vi "Modify CE template to Single point CE template.vi"(8 "error in (no error)":errorcluster, 10 "Measurement template file":path, 11 "SS measurement":T1 {"PJVS reference voltages array of vector cluster"."PJVS reference voltages vector" format="%#_3p"; "PJVS frequencies (Hz)" format="%#_3p"; "Record lengths (multiples of periods)" format="%#_3p"; "Sampling frequencies (Hz)" format="%#_3p"; "Signal amplitudes (V)" format="%#_3p"; "Signal frequencies (Hz)" format="%#_3p"}) -> (0 "error out":errorcluster)   [LabVIEW 2020]
doc: "Modify CE template - set CE measurement for only one frequency, sets amplitude and sampling frequency, removes possible previous measured data."
uses:
  SS Measurement/Type definitions/SS measurement.ctl
  <vilib>/Utility/NIReport.llb/Report Type.ctl
  <vilib>/Utility/NIReport.llb/NI_report.lvclass
  <vilib>/Utility/NIReport.llb/NI_ReportGenerationCore.lvlib
  external libraries/varilib/varilib.lvlib
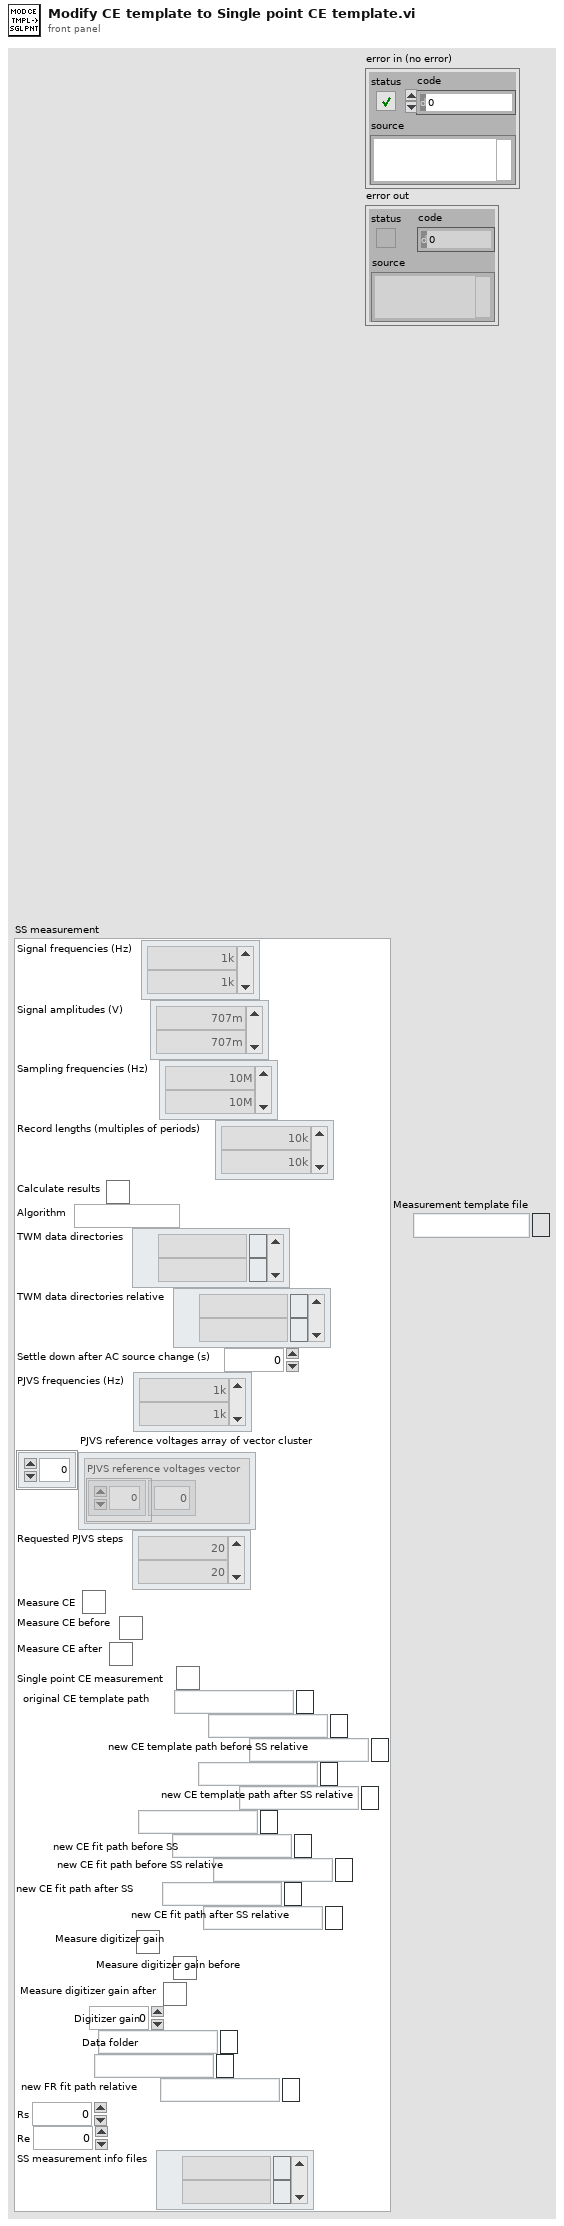
[diagram p1: front panel]
types:
  T1 = typedef "SS measurement.ctl" = cluster{"Signal frequencies (Hz)":dbl[], "Signal amplitudes (V)":dbl[], "Sampling frequencies (Hz)":dbl[], "Record lengths (multiples of periods)":dbl[], "Calculate results":bool, "Algorithm":string, "TWM data directories":path[], "TWM data directories relative":path[], "Settle down after AC source change (s)":dbl, "PJVS frequencies (Hz)":dbl[], "PJVS reference voltages array of vector cluster":cluster{"PJVS reference voltages vector":dbl[]}[], "Requested PJVS steps":u32[], "Measure CE":bool, "Measure CE before":bool, "Measure CE after":bool, "Single point CE measurement":bool, "original CE template path":path, "new CE template path before SS":path, "new CE template path before SS relative":path, "new CE template path after SS":path, "new CE template path after SS relative":path, "original CE fit path":path, "new CE fit path before SS":path, "new CE fit path before SS relative":path, "new CE fit path after SS":path, "new CE fit path after SS relative":path, "Measure digitizer gain":bool, "Measure digitizer gain before":bool, "Measure digitizer gain after":bool, "Digitizer gain":dbl, "Data folder":path, "FR fit path":path, "new FR fit path relative":path, "Rs":i32, "Re":i32, "SS measurement info files":path[]}
  T2 = typedef "NI_ReportGenerationCore.lvlib/Report Type.ctl" = enum16{"HTML", "Word", "Excel"}
  T3 = enum16{"maximized", "minimized", "normal", "no change"}
  T4 = typedef "Type definitions to be saved.ctl" = cluster{"Common properties":T5, "AC Source":T6, "DC meter":T8, "CE measurement":T10, "FR measurement":T11, "FR template":T12, "CE template":T13, "PJVS":T14, "SS measurement":T1, "AC sync source":T6}
  T5 = typedef "Common properties.ctl" = cluster{"Measurement status ref":refnum<vi>, "TWM Status ref":refnum<vi>, "Abort ref":refnum<vi>, "Skip waiting ref":refnum<vi>, "GNU Octave path":path, "TWM+QWTB path":path, "lvlib path":path, "TWM pipe":string, "PJVS status ref":refnum<vi>, "WAC path":path}
  T6 = typedef "AC Source.ctl" = cluster{"AC Source type":T7, "VISA":refnum<visa-resource-name>, "Ref. clock (Hz)":dbl, "status ref":refnum<vi>, "Fluke 57XX wideband output":bool, "Fluke 57XX ignore errors":bool, "Synchronization by AC signal":bool}
  T7 = typedef "AC Source type.ctl" = enum16{"Fluke 5XXX calibrator", "Tektronix AFG3000 series", "dummy", "Agilent 331xxA to 332xxA", "Agilent 335xxA to 336xxA"}
  T8 = typedef "DC meter.ctl" = cluster{"DC meter type":T9, "DC meter VISA":refnum<visa-resource-name>, "NPLC":dbl, "status ref":refnum<vi>}
  T9 = typedef "DC meter type.ctl" = enum16{"H/A/K 3458", "Fluke 8508A", "dummy", "Keithley 2182"}
  T10 = typedef "CE measurement.ctl" = cluster{"Signal frequencies (Hz) T":dbl[], "Signal amplitudes (V) T":dbl[], "Sampling frequencies (Hz) T":dbl[], "Record lengths (multiples of periods) T":dbl[], "TWM data root directory":path, "TWM mreasurements directories":path[], "Calculate RMS from samples":bool, "RMS algorithm T":string, "Settle down after AC source change (s) T":dbl, "Skip PJVS setup":bool, "Measurement template file":path, "Row of START keyword T":i32, "Row of STOP keyword T":i32, "Measurement template line T":i32[], "Switch position T":dbl[], "FR fit mat file T":path, "Recalculate-skip already calculated":bool}
  T11 = typedef "FR measuement.ctl" = cluster{"Measurement frequencies (Hz)":dbl[], "Sampling frequency (Hz)":dbl, "Signal amplitude (V)":dbl, "AC-DC settle time (s)":dbl, "Record length (multiples of period)":dbl[], "Measurement template file":path, "Row of START keyword":i32, "Row of STOP keyword":i32, "Calculate RMS from samples":bool, "AC-DC warm up time (s)":dbl, "Measurement template line":i32[], "DC meter readings No.":i32, "Algorithm":string, "Simultaneous measurement":bool, "Recalculate-skip already calculated":bool}
  T12 = typedef "FR template.ctl" = cluster{"Keywords column":i32, "Sig. freq. column":i32, "Rec. len. column":i32, "Meas. points. row min to read":i32, "Meas. points. row max to read":i32, "Properties column":i32, "Properties row start":i32, "Properties row end":i32, "Keyword START regexp":string, "Keyword STOP regexp":string, "HW data column":i32, "HW data row start":i32, "HW data row end":i32, "TIme and date column start":i32, "Digitizer value column start ":i32, "DC mean column start ":i32, "DC readings column start":i32}
  T13 = typedef "CE template.ctl" = cluster{"Keywords column":i32, "Sig. freq. column":i32, "Rec. len. column":i32, "Switch pos column":i32, "Meas. points. row min to read":i32, "Meas. points. row max to read":i32, "Properties column":i32, "Properties row start":i32, "Properties row end":i32, "Keyword START regexp":string, "Keyword STOP regexp":string, "HW data column":i32, "HW data row start":i32, "HW data row end":i32, "TIme and date column start":i32, "Digitizer value column start ":i32}
  T14 = typedef "PJVS.ctl" = cluster{"PJVS type":T15, "Status Refnum":refnum<vi>, "AC-supraVOLTcontrol":cluster{"IP address:port (0.0.0.0:0000)":string, "Timeouts":T16, "Simulation mode":bool, "Debug mode":bool}, "NPL bias source":cluster{"DataSocketCluster":T17}, "Manual PJVS":cluster{"PJVS frequency (Hz)":dbl, "Reference voltages (V)":dbl[], "File with PJVS voltages":path}, "VTT PJVS":cluster{"some VTT only property":string}}
  T15 = typedef "PJVS Type.ctl" = enum16{"AC-supraVOLTcontrol", "JV modified NPL bias control", "Manual PJVS", "VTT PJVS"}
  T16 = typedef "ACSVcontrol-driver.lvlib/Timeouts.ctl" = cluster{"TCP Read & Write (ms)":i32, "Sensors readout":i32, "PJVS setup":i32, "Nullmeter readout":i32, "Multiplexer setup":i32, "57XX setup":i32, "Generator setup":i32, "Synthesizer setup":i32, "Sampler readout":i32}
  T17 = typedef "DataSocketCluster external.ctl" = cluster{"Server Machine":string, "Client Machine":string, "Data":string, "TimeStamp":dbl, "Count":i32, "Target Process":string}
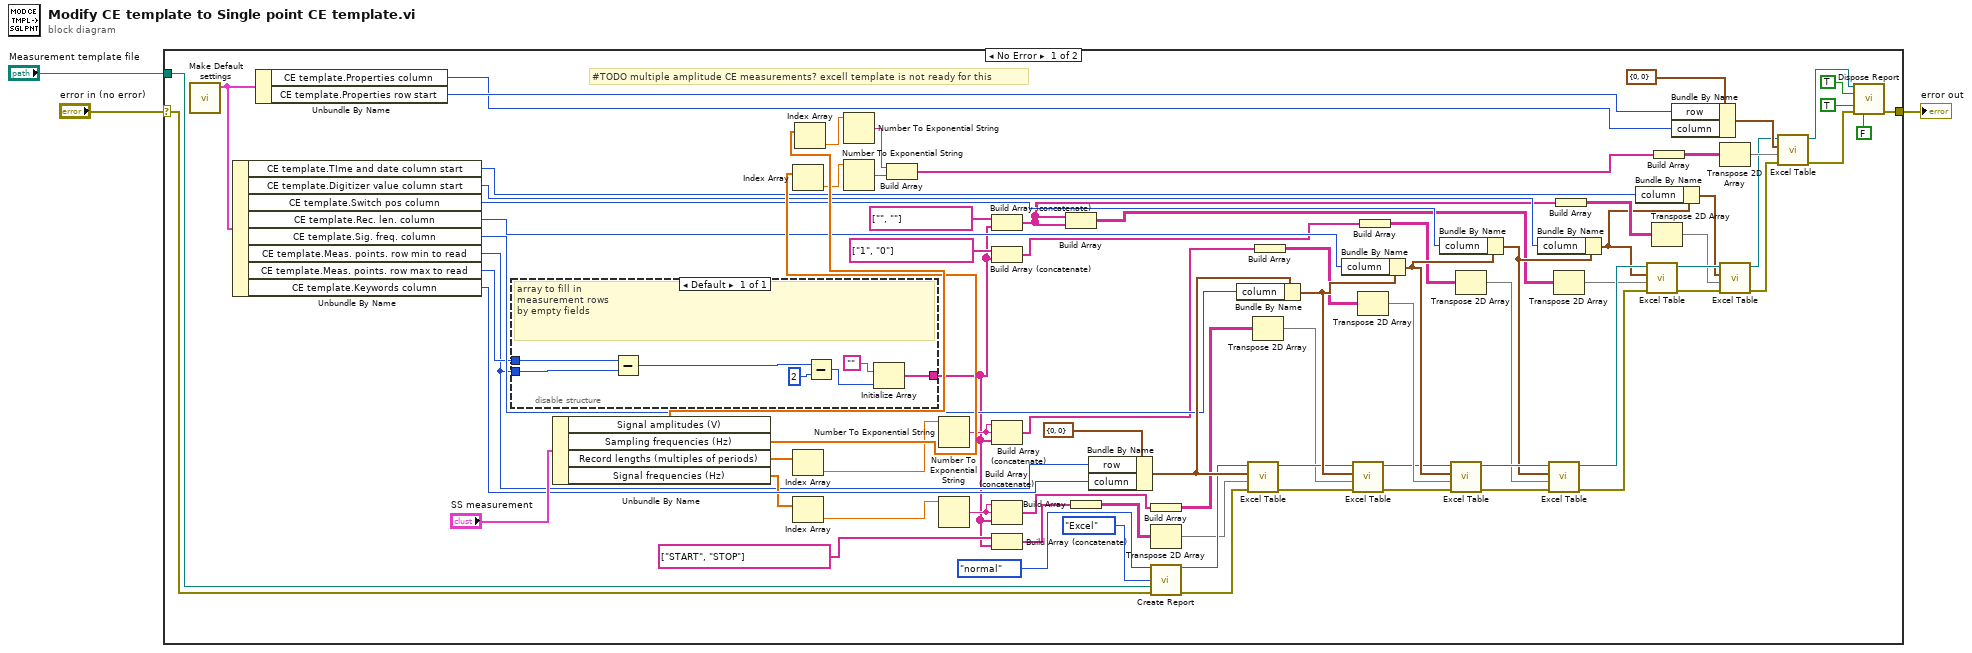
[diagram p0: block diagram]
diagram:
  n1 = case shown="No Error" "error in (no error)" {
    selector: "error in (no error)" -> [w46 w92]
    tunnel: [w49 w92] -> w3
    tunnel: "Measurement template file" -> [w5 _]
    frame No Error {
      # "#TODO multiple amplitude CE measurements? excell template is not ready for this"
      n2 = call "Make Default settings.vi"() -> ("TD to be saved"=w47:T4)  [unwired: 11 in]
      n3 = Unbundle By Name(w47) -> ("CE template.TIme and date column start"=w10:i32, "CE template.Digitizer value column start"=w11:i32, "CE template.Switch pos column"=w63:i32, "CE template.Rec. len. column"=w72:i32, "CE template.Sig. freq. column"=w64:i32, "CE template.Meas. points. row min to read"=w44:i32, "CE template.Meas. points. row max to read"=w45:i32, "CE template.Keywords column"=w65:i32)
      n4 = Unbundle By Name(w47) -> ("CE template.Properties column"=w26:i32, "CE template.Properties row start"=w27:i32)
      n5 = disable-structure shown="Default" {
        disable-tunnel: w45 -> [w90]
        disable-tunnel: w44 -> [w89]
        disable-tunnel: [w85] -> w24
        frame Enabled {
          # "array to fill in\nmeasurement rows \nby empty fields"
          n6 = Subtract(x=w90, y=w89) -> (x-y=w88:i32)
          n7 = Subtract(x=w88, y=2) -> (x-y=w86:i32)
          n8 = Initialize Array("", w86) -> (w85:string[])
        }
      }
      n9 = Unbundle By Name("SS measurement") -> ("Signal amplitudes (V)"=w83:dbl[], "Sampling frequencies (Hz)"=w82:dbl[], "Record lengths (multiples of periods)"=w81:dbl[], "Signal frequencies (Hz)"=w48:dbl[])
      n10 = Index Array(array=w82) -> (element=w59:dbl)  [unwired: 1 in]
      n11 = Index Array(array=w81) -> (element=w77:dbl)  [unwired: 1 in]
      n12 = Index Array(array=w48) -> (element=w78:dbl)  [unwired: 1 in]
      n13 = Index Array(array=w83) -> (element=w60:dbl)  [unwired: 1 in]
      n14 = Number To Exponential String(number=w60) -> (E-format string=w57:string)  [unwired: 3 in]
      n15 = Number To Exponential String(number=w59) -> (E-format string=w58:string)  [unwired: 3 in]
      n16 = Build Array(w57, w58) -> (w56:string[])
      n17 = Number To Exponential String(number=w77) -> (E-format string=w33:string)  [unwired: 3 in]
      n18 = Number To Exponential String(number=w78) -> (E-format string=w41:string)  [unwired: 3 in]
      n19 = Build Array (concatenate)(string[] ["", ""] ("appended array"), w24) -> (w9:string[])
      n20 = Build Array (concatenate)(string[] ["1", "0"] ("appended array"), w24) -> (w32:string[])
      n21 = Build Array (concatenate)(w33, w33, w24) -> (w35:string[])
      n22 = Build Array (concatenate)(w41, w41, w24) -> (w39:string[])
      n23 = Build Array (concatenate)(string[] ["START", "STOP"] ("appended array"), w24) -> (w40:string[])
      n24 = Build Array(w9, w9) -> (w8:string[][])
      n25 = Build Array(w40) -> (w28:string[][])
      n26 = Bundle By Name(cluster=cluster{"row":i32, "column":i32} {"row"=0, "column"=0} ("start (0, 0)"), "row"=w44, "column"=w65) -> (w75:cluster{"row":i32, "column":i32})
      n27 = Build Array(w39) -> (w38:string[][])
      n28 = Transpose 2D Array(2D array=w28) -> (transposed array=w42:string[][])
      n29 = call <vilib>:"Create Report.vi"("window state (normal)"=T3."normal", "report type"=Report_Type."Excel", "template (empty)"=w5, "error in (no error)"=w46) -> ("report out"=w68:refnum<class "NI_report.lvclass">, "error out"=w69:errorcluster)  [unwired: 10 in]
      n30 = Bundle By Name(cluster=w75, "column"=w64) -> (w73:cluster{"row":i32, "column":i32})
      n31 = call "Excel Table.vi"("error in (no error)"=w69, "table"=w42, "start (0, 0)"=w75, "report in"=w68) -> ("error out"=w74:errorcluster, "report out"=w67:refnum<class "NI_report.lvclass">)  [unwired: 6 in]
      n32 = Transpose 2D Array(2D array=w38) -> (transposed array=w37:string[][])
      n33 = Build Array(w35) -> (w36:string[][])
      n34 = Bundle By Name(cluster=w73, "column"=w72) -> (w70:cluster{"row":i32, "column":i32})
      n35 = call "Excel Table.vi"("error in (no error)"=w74, "table"=w37, "start (0, 0)"=w73, "report in"=w67) -> ("error out"=w20:errorcluster, "report out"=w19:refnum<class "NI_report.lvclass">)  [unwired: 6 in]
      n36 = Transpose 2D Array(2D array=w36) -> (transposed array=w34:string[][])
      n37 = Build Array(w32) -> (w31:string[][])
      n38 = Bundle By Name(cluster=w70, "column"=w63) -> (w14:cluster{"row":i32, "column":i32})
      n39 = call "Excel Table.vi"("error in (no error)"=w20, "table"=w34, "start (0, 0)"=w70, "report in"=w19) -> ("error out"=w71:errorcluster, "report out"=w66:refnum<class "NI_report.lvclass">)  [unwired: 6 in]
      n40 = Transpose 2D Array(2D array=w31) -> (transposed array=w29:string[][])
      n41 = Bundle By Name(cluster=w14, "column"=w11) -> (w13:cluster{"row":i32, "column":i32})
      n42 = call "Excel Table.vi"("error in (no error)"=w71, "table"=w29, "start (0, 0)"=w14, "report in"=w66) -> ("error out"=w18:errorcluster, "report out"=w17:refnum<class "NI_report.lvclass">)  [unwired: 6 in]
      n43 = Transpose 2D Array(2D array=w8) -> (transposed array=w7:string[][])
      n44 = Build Array(w9) -> (w23:string[][])
      n45 = Bundle By Name(cluster=w13, "column"=w10) -> (w12:cluster{"row":i32, "column":i32})
      n46 = call "Excel Table.vi"("error in (no error)"=w18, "table"=w7, "start (0, 0)"=w13, "report in"=w17) -> ("error out"=w22:errorcluster, "report out"=w21:refnum<class "NI_report.lvclass">)  [unwired: 6 in]
      n47 = Transpose 2D Array(2D array=w23) -> (transposed array=w6:string[][])
      n48 = Build Array(w56) -> (w55:string[][])
      n49 = Bundle By Name(cluster=cluster{"row":i32, "column":i32} {"row"=0, "column"=0} ("start (0, 0)"), "row"=w27, "column"=w26) -> (w62:cluster{"row":i32, "column":i32})
      n50 = Transpose 2D Array(2D array=w55) -> (transposed array=w54:string[][])
      n51 = call "Excel Table.vi"("error in (no error)"=w22, "table"=w6, "start (0, 0)"=w12, "report in"=w21) -> ("error out"=w15:errorcluster, "report out"=w16:refnum<class "NI_report.lvclass">)  [unwired: 6 in]
      n52 = call "Excel Table.vi"("error in (no error)"=w15, "table"=w54, "start (0, 0)"=w62, "report in"=w16) -> ("error out"=w51:errorcluster, "report out"=w52:refnum<class "NI_report.lvclass">)  [unwired: 6 in]
      n53 = call-dynamic "Dispose Report.vi"("report in"=w52, "wait until printing completed? (T)"=TRUE, "save changes? (F)"=TRUE, "error in (no error)"=w51, "close report? (T)"=FALSE) -> ("error out"=w49:errorcluster)  [unwired: 10 in]
    }
    frame Error {
    }
  }
  "error out" <- w3
